vi "adjustdacutil.vi"(4 "min":dbl, 5 "max":dbl, 6 "ori dac":dbl, 7 "work":bool, 9 "settings":T1, 11 "real":dbl) -> (0 "new max":dbl, 1 "dac":dbl, 2 "amplitude":dbl, 3 "ok":bool, 8 "new min":dbl)   [LabVIEW 2012]
panel:
  in  "algrithom":enum16{"step", "2divice"}(ring)
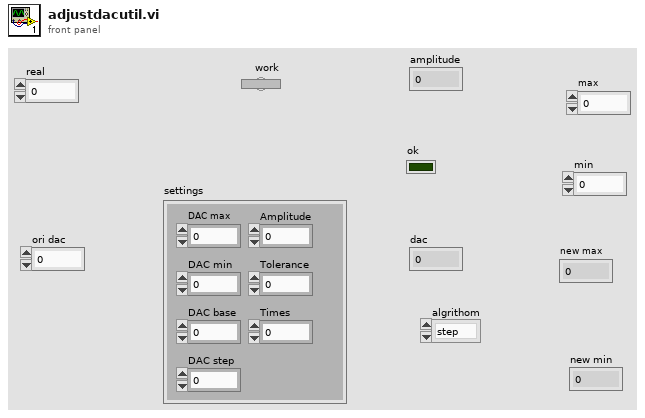
[diagram p1: front panel]
types:
  T1 = cluster{"DAC max":dbl, "DAC min":dbl, "DAC base":dbl, "DAC step":dbl, "Amplitude":dbl, "Tolerance":dbl, "Times":dbl}
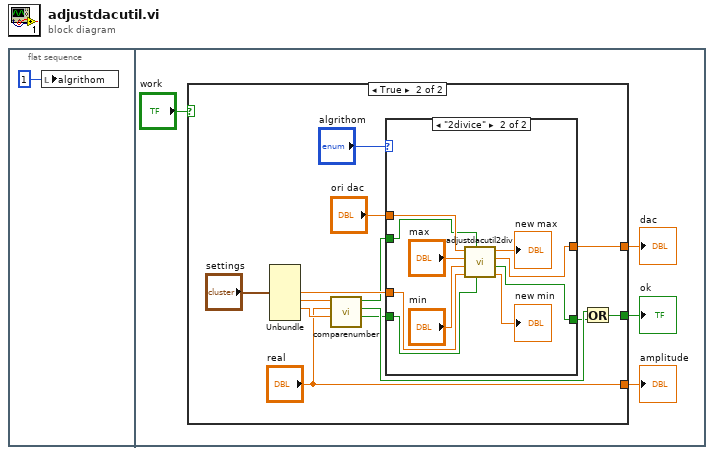
[diagram p0: block diagram]
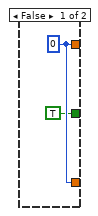
[diagram p2: hidden frame]
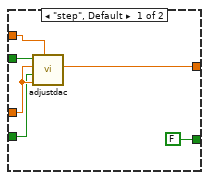
[diagram p3: hidden frame]
diagram:
  n1 = flat-sequence {
    frame #0 {
      n2 = local write "algrithom"(1) -> ()
    }
    frame #1 {
      n3 = case shown="True" "work" {
        tunnel: [TRUE w9] -> w5
        tunnel: [w7 w16] -> w4
        tunnel: [w7 "real"] -> w3
        frame False {
          w7 = 0
        }
        frame True {
          n4 = Unbundle("settings") -> ("DAC step"=w14:dbl, "Amplitude"=w19:dbl, "Tolerance"=w18:dbl)  [unwired: 4 out]
          n5 = call "comparenumber.vi"("limit adjust"=w18, "x"="real", "base"=w19) -> ("smaller"=w10:bool, "equal"=w13:bool, "bigger"=w11:bool)  [unwired: 6 in]
          n6 = case shown="\"2divice\"" "algrithom" {
            tunnel: [w26 w32] -> w16
            tunnel: "ori dac" -> [w25 w36]
            tunnel: w11 -> [w24 w35]
            tunnel: w14 -> [w23 w33]
            tunnel: w10 -> [w22 w34]
            tunnel: [FALSE w31] -> w12
            frame "step", Default {
              n7 = call "adjustdac.vi"("input"=w25, "down step"=w23, "increase"=w22, "up step"=w23, "decrease"=w24) -> ("output"=w26:dbl)  [unwired: 6 in]
            }
            frame "2divice" {
              n8 = call "adjustdacutil2div.vi"("smaller"=w34, "bigger"=w35, "step"=w33, "min dac"="min", "max dac"="max", "ori dac"=w36) -> ("new min"=→"new min":dbl, "no need"=w31:bool, "dac"=w32:dbl, "new max"=→"new max":dbl)  [unwired: 2 in]
            }
          }
          n9 = Or(x=w13, y=w12) -> (x .or. y?=w9:bool)
        }
      }
      "amplitude" <- w3
      "dac" <- w4
      "ok" <- w5
    }
  }
